vi "Ann_int.vi"(0 "Data":dbl[](array[numeric]), 1 "Loss Function":enum16{"MSE", "MAE"}(ring), 5 "Target":dbl format="%#_13g", 7 "Training?":bool, 9 "Parameters":T2, 13 "Adam Data In":T1) -> (4 "Output":dbl, 6 "Error":dbl, 10 "Adjusted Parameters":T2, 14 "Adam Data Out":T1)   [LabVIEW 2018]
uses:
  Sub-VI's/Adam_data.ctl
  Sub-VI's/Globals.vi
  Sub-VI's/Layer.vi
  Sub-VI's/Layer1d.vi
panel:
  out "Error Codes":i32[](array[numeric])
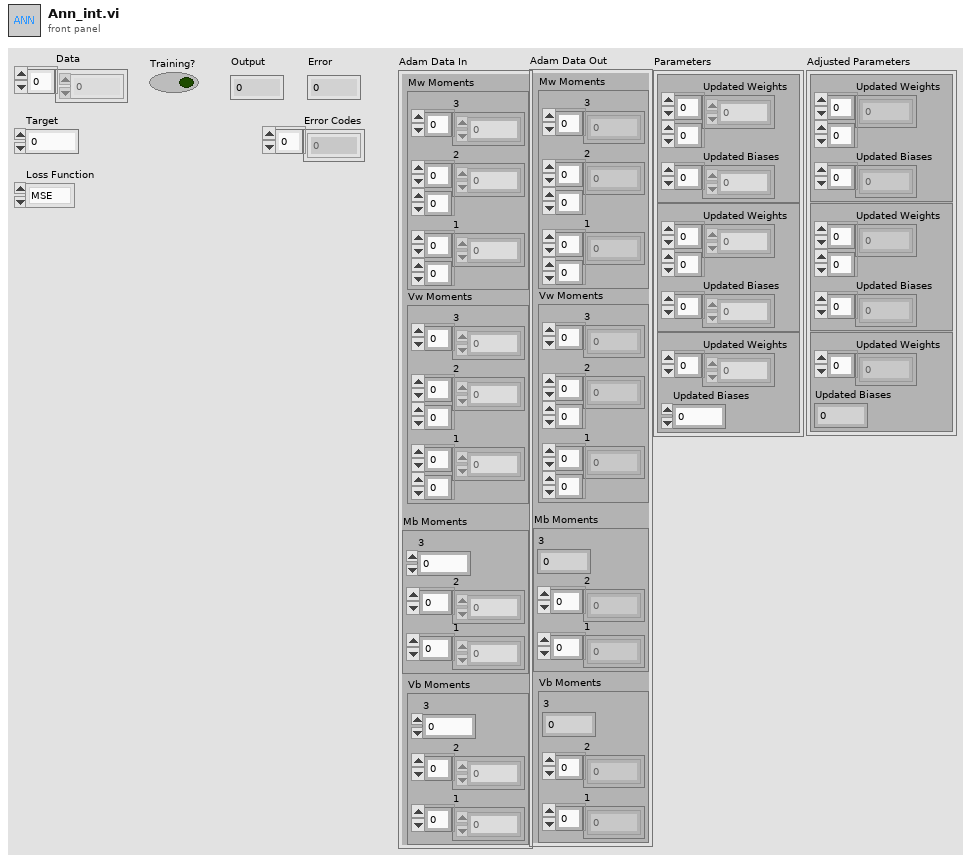
[diagram p1: front panel]
types:
  T1 = typedef "Adam_data.ctl" = cluster{"Mw Moments":cluster{"3 ":dbl[], "2":dbl[][], "1":dbl[][]}, "Vw Moments":cluster{"3":dbl[], "2":dbl[][], "1":dbl[][]}, "Mb Moments":cluster{"3":dbl, "2":dbl[], "1":dbl[]}, "Vb Moments":cluster{"3":dbl, "2":dbl[], "1":dbl[]}}
  T2 = cluster{cluster{"Updated Weights":dbl[][], "Updated Biases":dbl[]}, cluster{"Updated Weights":dbl[][], "Updated Biases":dbl[]}, cluster{"Updated Weights":dbl[], "Updated Biases":dbl}}
  T3 = cluster{"Updated Weights":dbl[][], "Updated Biases":dbl[]}
  T4 = cluster{"Updated Weights":dbl[], "Updated Biases":dbl}
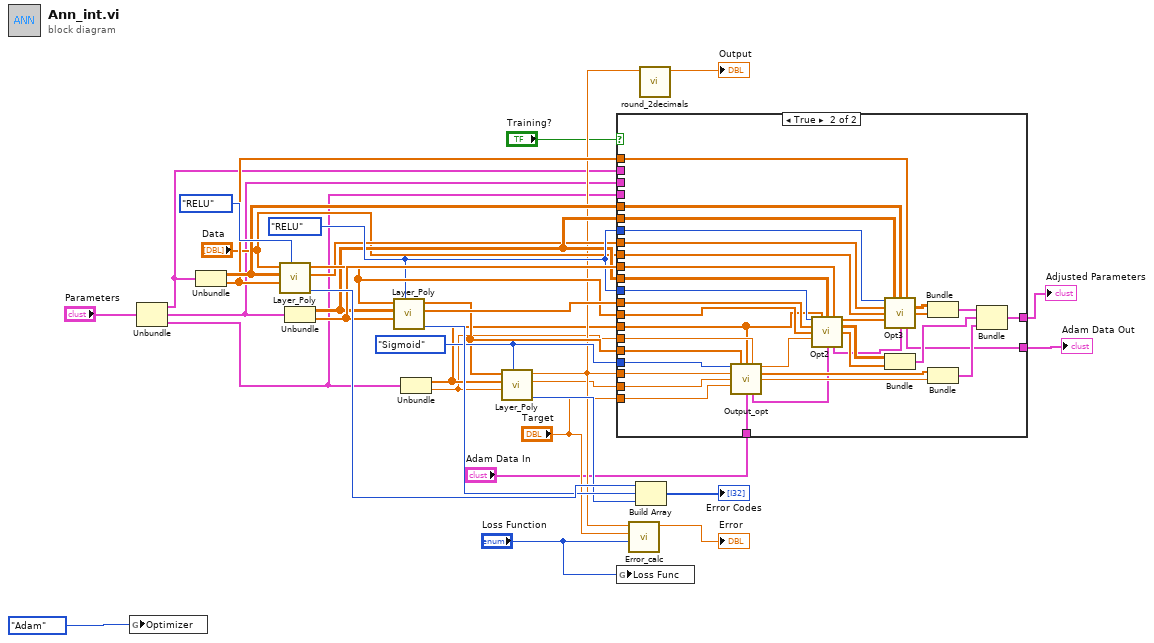
[diagram p0: block diagram]
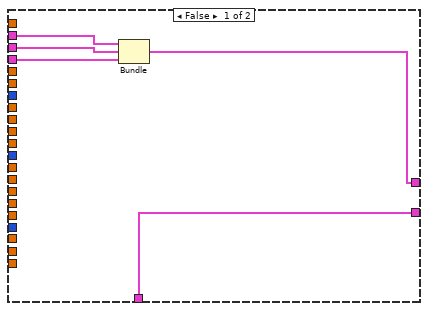
[diagram p2: hidden frame]
diagram:
  w17 = enum32{"Sigmoid", "RELU", "Tanh", "Leaky RELU"}."Sigmoid" ("Activation Function")
  w23 = enum32{"Sigmoid", "RELU", "Tanh", "Leaky RELU"}."RELU" ("Activation Function")
  n1 = global write "Globals.vi" "Optimizer"(enum16{"Adagrad", "Adadelta", "Adam"}."Adam" ("Optimizer")) -> ()
  n2 = Unbundle("Parameters") -> (w12:T3, w11:T3, w10:T4)
  n3 = Unbundle(w12) -> ("Updated Weights"=w21:dbl[][], "Updated Biases"=w20:dbl[])
  n4 = call-poly "Layer_Poly.vi"("Activation Function"=enum32{"Sigmoid", "RELU", "Tanh", "Leaky RELU"}."RELU", "Biases"=w20, "Weights"=w21, "Data"="Data") -> ("Error"=w32:i32, "Net Activation"=w19:dbl[], "Output"=w24:dbl[])  [unwired: 5 in]
  n5 = Unbundle(w11) -> ("Updated Weights"=w22:dbl[][], "Updated Biases"=w26:dbl[])
  n6 = call-poly "Layer_Poly.vi"("Activation Function"=w23, "Biases"=w26, "Weights"=w22, "Data"=w24) -> ("Error"=w31:i32, "Net Activation"=w25:dbl[], "Output"=w16:dbl[])  [unwired: 5 in]
  n7 = Unbundle(w10) -> ("Updated Weights"=w9:dbl[], "Updated Biases"=w8:dbl)
  n8 = call-poly "Layer_Poly.vi"("Activation Function"=w17, "Biases"=w8, "Weights"=w9, "Data"=w16) -> ("Error"=w30:i32, "Net Activation"=w14:dbl, "Output"=w15:dbl)  [unwired: 5 in]
  n9 = case shown="True" "Training?" {
    tunnel: w23 -> [_ w72]
    tunnel: w22 -> [_ w71]
    tunnel: w26 -> [_ w70]
    tunnel: w25 -> [_ w69]
    tunnel: w24 -> [_ w68]
    tunnel: w23 -> [_ w67]
    tunnel: w22 -> [_ w66]
    tunnel: w21 -> [_ w65]
    tunnel: w20 -> [_ w64]
    tunnel: w19 -> [_ w63]
    tunnel: "Data" -> [_ w62]
    tunnel: w17 -> [_ w60]
    tunnel: w16 -> [_ w59]
    tunnel: w15 -> [_ w58]
    tunnel: w14 -> [_ w57]
    tunnel: "Target" -> [_ w56]
    tunnel: [w35 w41] -> w1
    tunnel: w12 -> [w38 _]
    tunnel: w11 -> [w37 _]
    tunnel: w10 -> [w36 _]
    tunnel: w9 -> [_ w48]
    tunnel: w8 -> [_ w49]
    tunnel: [w34 w40] -> w4
    tunnel: "Adam Data In" -> [w34 w39]
    frame False {
      n10 = Bundle(w38, w37, w36) -> (w35:T2)  [unwired: 1 in]
    }
    frame True {
      n11 = call "Output_opt.vi"("Activation Function"=w60, "Activation l-1"=w59, "Weights"=w48, "Biases"=w49, "Activation"=w58, "Net Output"=w57, "Target"=w56, "Adam Data In"=w39) -> ("Delta"=w55:dbl, "Updated Weights"=w52:dbl[], "Updated Biases"=w51:dbl, "Adam Data Out"=w43:T1)  [unwired: 4 in]
      n12 = call "Opt2.vi"("Activation Function"=w72, "Weights l+1"=w48, "Weights"=w71, "Biases"=w70, "Net Output"=w69, "Activations l-1"=w68, "Delta l+1"=w55, "Adam Data In"=w43) -> ("Delta l"=w61:dbl[], "Updated Weights"=w47:dbl[][], "Updated Biases"=w46:dbl[], "Adam Data Out"=w42:T1)  [unwired: 4 in]
      n13 = call "Opt3.vi"("Activation Function"=w67, "Weights l+1"=w66, "Weights"=w65, "Biases"=w64, "Net Output"=w63, "Activations l-1"=w62, "Delta l+1"=w61, "Adam Data In"=w42) -> ("Updated Weights"=w45:dbl[][], "Updated Biases"=w44:dbl[], "Adam Data Out"=w40:T1)  [unwired: 5 in]
      n14 = Bundle("Updated Weights"=w47, "Updated Biases"=w46) -> (w54:T3)  [unwired: 1 in]
      n15 = Bundle("Updated Weights"=w45, "Updated Biases"=w44) -> (w53:T3)  [unwired: 1 in]
      n16 = Bundle("Updated Weights"=w52, "Updated Biases"=w51) -> (w50:T4)  [unwired: 1 in]
      n17 = Bundle(w53, w54, w50) -> (w41:T2)  [unwired: 1 in]
    }
  }
  "Adjusted Parameters" <- w1
  "Adam Data Out" <- w4
  n18 = global write "Globals.vi" "Loss Func"("Loss Function") -> ()
  n19 = call "Error_calc.vi"("Error Type"="Loss Function", "Target"="Target", "Data"=w15) -> ("Error"=→"Error":dbl)  [unwired: 8 in]
  n20 = Build Array(w32, w31, w30) -> (→"Error Codes":i32[])
  n21 = call "round_2decimals.vi"("Number"=w15) -> ("Rounded Number"=→"Output":dbl)  [unwired: 10 in]
